vi "FTW-JSON-LexicalScan-Digit.vi"(0 "JSON String":T1, 11 "error in":errorcluster) -> (4 "JSON String Out":T1, 8 "Digits":u64, 15 "error out":errorcluster)   [LabVIEW 2015]
uses:
  FTW-JSON-LexicalScan.ctl
panel:
  # "Inputs"
  # "Outputs"
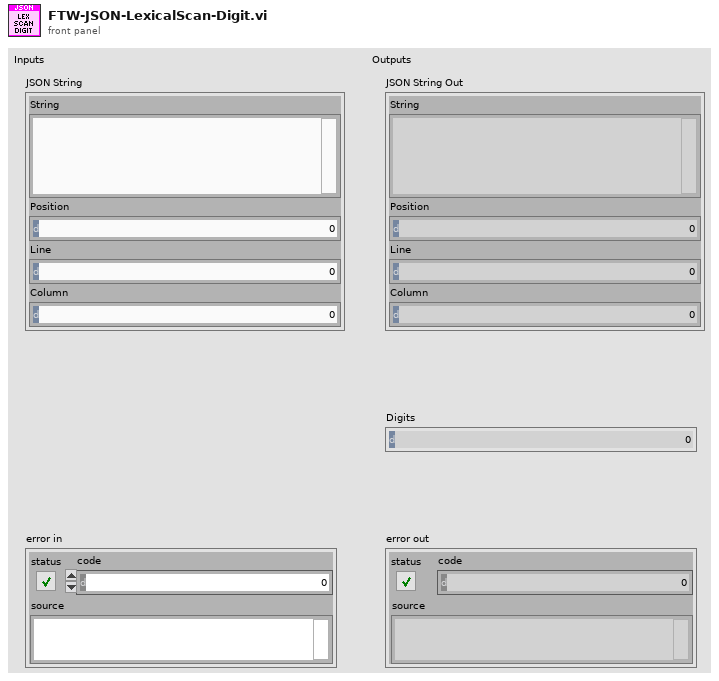
[diagram p1: front panel]
types:
  T1 = typedef "FTW-JSON-LexicalScan.ctl" = cluster{"String":string, "Position":i32, "Line":i32, "Column":i32}
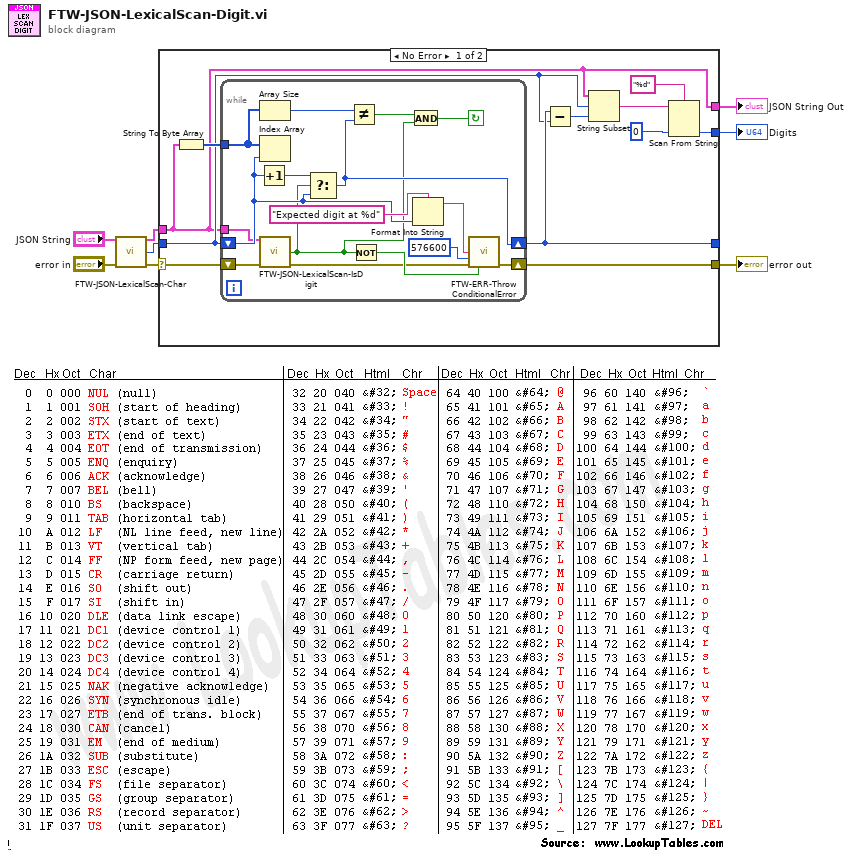
[diagram p0: block diagram]
diagram:
  n1 = call "FTW-JSON-LexicalScan-Char.vi"("JSON String"="JSON String", "error in"="error in") -> ("JSON String Out"=w2:T1, "Char"=w1:u8, "error out"=w4:errorcluster)  [unwired: 11 in]
  n2 = case shown="No Error" w4 {
    selector: w4 -> [w17 w38]
    tunnel: w1 -> [w12 w37]
    tunnel: w2 -> [w9 w36]
    tunnel: [w19 w38] -> w8
    tunnel: [w13 w37] -> _
    tunnel: [w14 _] -> w6
    tunnel: [w9 w36] -> w5
    frame No Error {
      n3 = String To Byte Array(string=w9) -> (unsigned byte array=w18:u8[])
      n4 = while {
        tunnel: w18 -> [w28]
        shift-right: [w26] -> w13
        shift-left: w12 -> [w29]
        shift-right: [w35] -> w19
        shift-left: w17 -> [w23]
        tunnel: w9 -> [w21]
        stop <- w25 continue-if-true
        n5 = Increment(x=w29) -> (x+1=w30:u8)
        n6 = Array Size(array=w28) -> (size(s)=w27:i32)
        n7 = Index Array(array=w28, index=w29) -> ()  [unwired: 1 out]
        n8 = call "FTW-JSON-LexicalScan-IsDigit.vi"("JSON String"=w21, "error in"=w23) -> ("Is Digit"=w20:bool, "error out"=w22:errorcluster)  [unwired: 11 in, 1 out]
        n9 = Select(t=w30, s=w20, f=w29) -> (s? t:f=w26:u8)
        n10 = Not Equal?(x=w27, y=w26) -> (x != y?=w24:bool)
        n11 = Not(x=w20) -> (.not. x?=w31:bool)
        n12 = And(x=w24, y=w20) -> (x .and. y?=w25:bool)
        n13 = Format Into String(format string="Expected digit at %d" ("Error Message"), w29) -> (resulting string=w32:string)  [unwired: 2 in, 1 out]
        n14 = call "FTW-ERR-ThrowConditionalError.vi"("Error Message"=w32, "Error Code"=576600, "error in"=w22, "Throw Error?"=w31) -> ("error out"=w35:errorcluster)  [unwired: 11 in]
      }
      n15 = Subtract(x=w13, y=w12) -> (x-y=w11:u8)
      n16 = String Subset(string=w9, offset (0)=w12, length (rest)=w11) -> (substring=w10:string)
      n17 = Scan From String(format string="%d", input string=w10, default 1=u64 0 ("default value 1")) -> (output 1=w14:u64)  [unwired: 2 in, 3 out]
    }
    frame Error {
    }
  }
  "Digits" <- w6
  "error out" <- w8
  "JSON String Out" <- w5
